vi "main_4.vi"(11 "error in (no error)":errorcluster) -> (15 "error out":errorcluster)   [LabVIEW 2023, in "task_4.lvlib"]
doc: "Open www.solitontech.com on chrome"
uses:
  task_4.lvlib
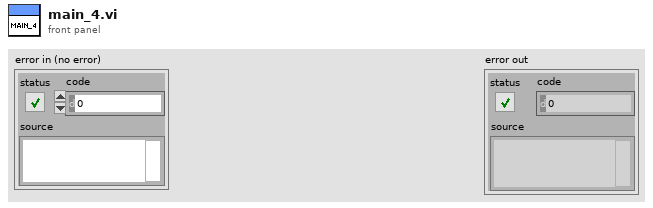
[diagram p1: front panel]
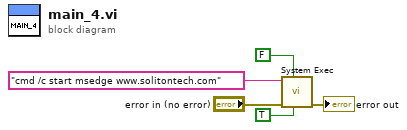
[diagram p0: block diagram]
diagram:
  n1 = call <vilib>:"System Exec.vi"("run minimized? (F)"=TRUE, "wait until completion? (T)"=FALSE, "error in (no error)"="error in (no error)", "command line"="cmd /c start msedge www.solitontech.com") -> ("error out"=→"error out":errorcluster)  [unwired: 4 in, 3 out]
